vi "FT_Purge_64bit.vi"(3 "error in (no error)":errorcluster, 4 "Purge Flags":u32(ring)=3 items=["FT_PURGE_RX"=1, "FT_PURGE_TX"=2, "FT_PURGE_RX | FT_PURGE_TX"=3], 5 "Handle in":u64) -> (0 "error out":errorcluster, 1 "FT_Status":u32(ring) items=["FT_OK", "FT_INVALID_HANDLE", "FT_DEVICE_NOT_FOUND", "FT_DEVICE_NOT_OPENED", "FT_IO_ERROR", "FT_INSUFFICIENT_RESOURCES", "FT_INVALID_PARAMETER", "FT_INVALID_BAUD_RATE", "FT_DEVICE_NOT_OPENED_FOR_ERASE", "FT_DEVICE_NOT_OPENED_FOR_WRITE", "FT_FAILED_TO_WRITE_DEVICE", "FT_EEPROM_READ_FAILED", "FT_EEPROM_WRITE_FAILED", "FT_EEPROM_ERASE_FAILED", "FT_EEPROM_NOT_PRESENT", "FT_EEPROM_NOT_PROGRAMMED", "FT_INVALID_ARGS", "FT_NOT_SUPPORTED", "FT_OTHER_ERROR"], 2 "Handle Out":u64)   [LabVIEW 2019]
uses:
  FTD2XX.dll
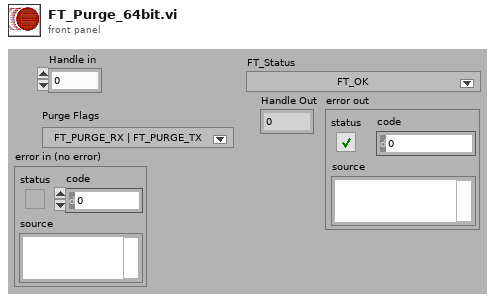
[diagram p1: front panel]
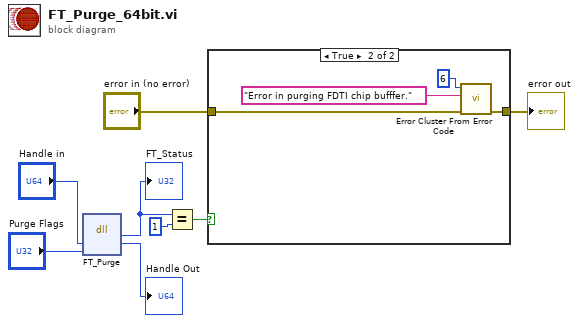
[diagram p0: block diagram]
diagram:
  n1 = dll-call lib="FTD2XX.dll" fn="FT_Purge"("Handle"="Handle in", "Flags"="Purge Flags") -> ("FT_Status"=w5:u32, "Handle"=→"Handle Out":u64)  [unwired: 4 in, 2 out]
  "FT_Status" <- w5
  n2 = Equal?(x=w5, y=u32 1) -> (x = y?=w6:bool)
  n3 = case shown="True" w6 {
    tunnel: [w9 w12] -> w1
    tunnel: "error in (no error)" -> [w9 w11]
    frame False {
    }
    frame True {
      n4 = call <vilib>:"Error Cluster From Error Code.vi"("error in (no error)"=w11, "error message (\"\")"="Error in purging FDTI chip bufffer." ("error message (\"\")"), "error code (0)"=6) -> ("error out"=w12:errorcluster)  [unwired: 6 in]
    }
  }
  "error out" <- w1
